vi "Calculate framerate.vi"(6 "Time at start of save":u32, 7 "# saved frames in":i32, 9 "Saving File":bool, 10 "frame rate var in":i32, 11 "tick var":u32) -> (1 "Rate Hz":dbl, 2 "Tick var out":u32, 3 "Frame rate var out":i32, 4 "# saved frames out":i32)   [LabVIEW 2011]
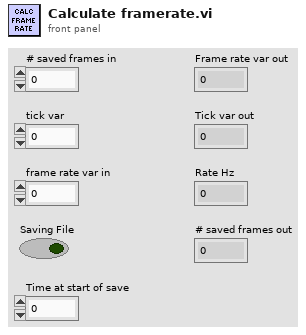
[diagram p1: front panel]
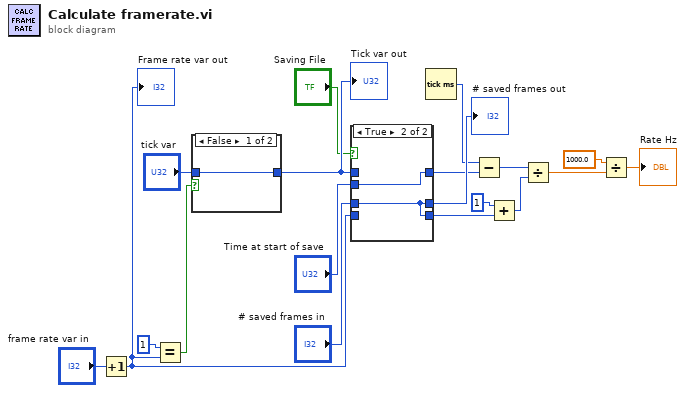
[diagram p0: block diagram]
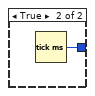
[diagram p3: hidden frame]
diagram:
  n1 = Increment(x="frame rate var in") -> (x+1=w17:i32)
  "Frame rate var out" <- w17
  n2 = Equal?(x=1, y=w17) -> (x = y?=w10:bool)
  n3 = case shown="False" w10 {
    tunnel: [w20 w21] -> w16
    tunnel: "tick var" -> [w20 _]
    frame False {
    }
    frame True {
      n4 = Tick Count (ms)() -> (millisecond timer value=w21:u32)
    }
  }
  "Tick var out" <- w16
  n5 = case shown="True" "Saving File" {
    tunnel: "Time at start of save" -> [_ w26]
    tunnel: [w24 w26] -> w13
    tunnel: "# saved frames in" -> [w22 w25]
    tunnel: [w23 w25] -> w15
    tunnel: w16 -> [w24 _]
    tunnel: w17 -> [w23 _]
    tunnel: [w22 w25] -> w18
    frame False {
    }
    frame True {
    }
  }
  "# saved frames out" <- w18
  n6 = Tick Count (ms)() -> (millisecond timer value=w7:u32)
  n7 = Subtract(x=w7, y=w13) -> (x-y=w3:u32)
  n8 = Add(x=1, y=w15) -> (x+y=w1:i32)
  n9 = Divide(x=w3, y=w1) -> (x/y=w5:dbl)
  n10 = Divide(x=1000.0, y=w5) -> (x/y=→"Rate Hz":dbl)
